vi "To Pretty String (Object).vi"(0 "Variant in":variant, 5 "indent":i32, 7 "enable LabVIEW extensions? (T)":bool=TRUE, 9 "pretty print? (T)":bool=TRUE, 11 "error in (no error)":errorcluster) -> (4 "Pretty Print String":string, 15 "error out":errorcluster)   [LabVIEW 2017, in "Advanced Variant Tools.lvlib"]
doc: "Pretty prints the given JSON data in an easier to read format."
uses:
  Advanced Variant Tools.lvlib
  <vilib>/National Instruments/Variant Data Manipulation/Variant Data Manipulation.lvlib
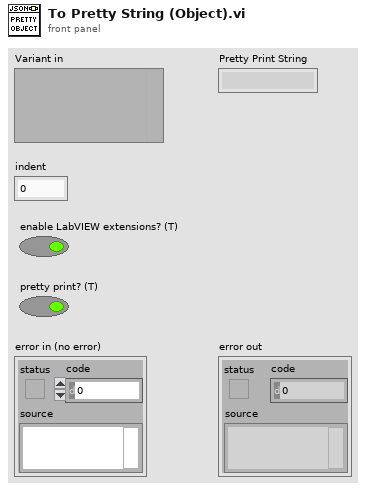
[diagram p1: front panel]
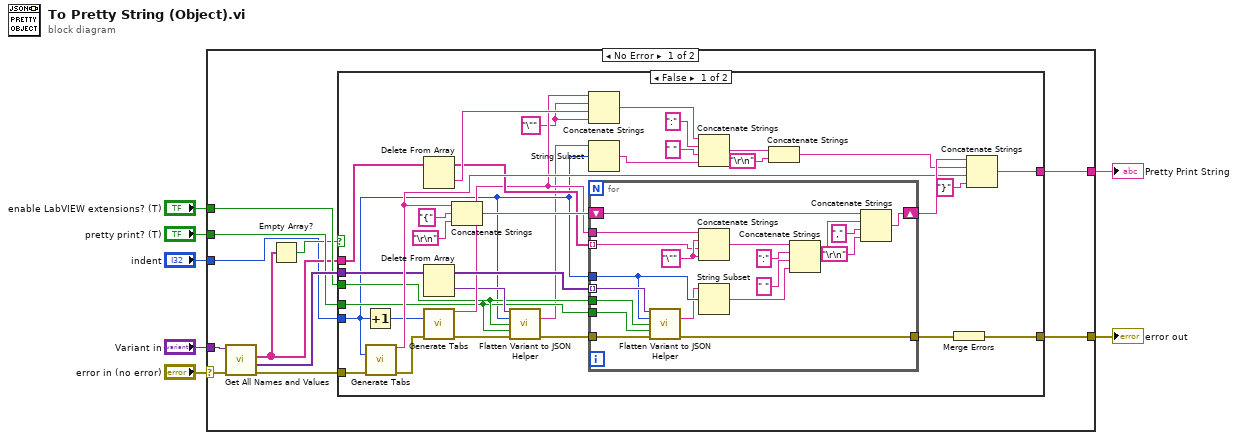
[diagram p0: block diagram]
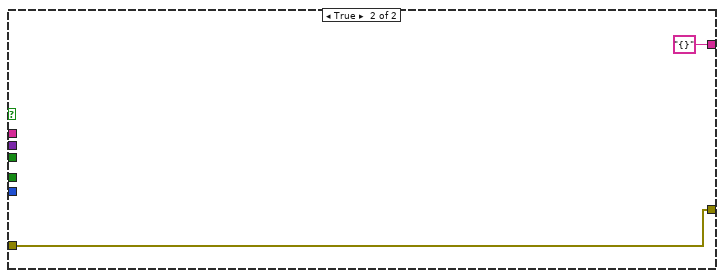
[diagram p2: hidden frame]
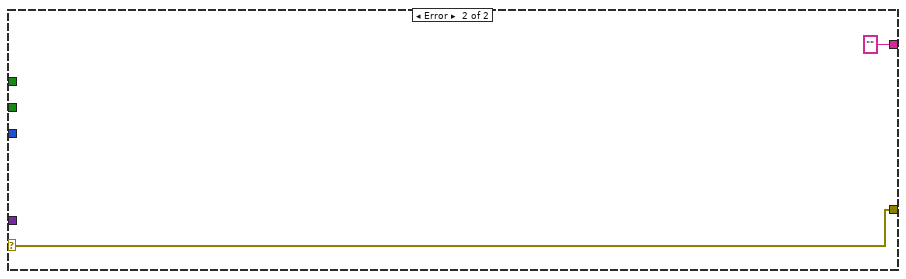
[diagram p3: hidden frame]
diagram:
  n1 = case shown="No Error" "error in (no error)" {
    selector: "error in (no error)" -> [w9 w73]
    tunnel: [w18 ""] -> w7
    tunnel: [w17 w73] -> w6
    tunnel: "Variant in" -> [w15 _]
    tunnel: "enable LabVIEW extensions? (T)" -> [w14 _]
    tunnel: "pretty print? (T)" -> [w13 _]
    tunnel: "indent" -> [w10 _]
    frame No Error {
      n2 = call <vilib>:"Get All Names and Values.vi"("error in"=w9, "Cluster in"=w15) -> ("error out"=w8:errorcluster, "Values"=w16:variant[], "Element Names"=w11:string[])  [unwired: 5 in, 2 out]
      n3 = Empty Array?(array=w11) -> (empty?=w12:bool)
      n4 = case shown="False" w12 {
        tunnel: [w42 "{}"] -> w18
        tunnel: [w49 w71] -> w17
        tunnel: w8 -> [w41 w71]
        tunnel: w16 -> [w40 _]
        tunnel: w14 -> [w32 _]
        tunnel: w13 -> [w31 _]
        tunnel: w11 -> [w30 _]
        tunnel: w10 -> [w20 _]
        frame False {
          w26 = "\"" ("string")
          n5 = Increment(x=w20) -> (x+1=w22:i32)
          n6 = call "Generate Tabs.vi"("indent"=w20, "error in (no error)"=w41) -> ("Tabs"=w43:string, "error out"=w29:errorcluster)  [unwired: 12 in]
          n7 = Delete From Array(array=w30) -> (deleted portion=w39:string, array with subset deleted=w38:string[])  [unwired: 2 in]
          n8 = Delete From Array(array=w40) -> (deleted portion=w35:variant, array with subset deleted=w48:variant[])  [unwired: 2 in]
          n9 = call "Generate Tabs.vi"("indent"=w22, "error in (no error)"=w29) -> ("Tabs"=w37:string, "error out"=w34:errorcluster)  [unwired: 12 in]
          n10 = Concatenate Strings(w43, "{" ("string"), "\r\n") -> (w50:string)
          n11 = call "Flatten Variant to JSON Helper.vi"("Variant in"=w35, "indent"=w20, "enable LabVIEW extensions? (T)"=w32, "pretty print? (T)"=w31, "error in (no error)"=w34) -> ("String"=w19:string, "error out"=w33:errorcluster)  [unwired: 8 in, 1 out]
          n12 = Concatenate Strings(w37, w26, w39, w26) -> (w25:string)
          n13 = String Subset(string=w19, offset (0)=w20) -> (substring=w21:string)  [unwired: 1 in]
          n14 = for {
            tunnel: w48 -> [w58] mode=indexing
            shift-right: [w68] -> w47
            shift-left: w50 -> [w67]
            tunnel: w37 -> [w60]
            tunnel: w38 -> [w63] mode=indexing
            tunnel: w33 -> [w59]
            tunnel: [w57] -> w36
            tunnel: w32 -> [w56]
            tunnel: w31 -> [w55]
            tunnel: w20 -> [w53]
            w65 = "\"" ("string")
            n15 = call "Flatten Variant to JSON Helper.vi"("Variant in"=w58, "indent"=w53, "enable LabVIEW extensions? (T)"=w56, "pretty print? (T)"=w55, "error in (no error)"=w59) -> ("String"=w52:string, "error out"=w57:errorcluster)  [unwired: 8 in, 1 out]
            n16 = Concatenate Strings(w60, w65, w63, w65) -> (w66:string)
            n17 = String Subset(string=w52, offset (0)=w53) -> (substring=w54:string)  [unwired: 1 in]
            n18 = Concatenate Strings(w66, ":" ("string"), " " ("string"), w54) -> (w62:string)
            n19 = Concatenate Strings(w67, w62, "," ("string"), "\r\n") -> (w68:string)
          }
          n20 = Concatenate Strings(w25, ":" ("string"), " " ("string"), w21) -> (w24:string)
          n21 = Concatenate Strings(w24, "\r\n") -> (w46:string)
          n22 = Merge Errors(w36) -> (w49:errorcluster)
          n23 = Concatenate Strings(w47, w46, w43, "}" ("string")) -> (w42:string)
        }
        frame True {
        }
      }
    }
    frame Error {
    }
  }
  "error out" <- w6
  "Pretty Print String" <- w7
